vi "Cashew Model.vi"() -> ()   [LabVIEW 2018]
uses:
  <vilib>/express/express arith-compare/Formula/XNode/ExpressFormulaBlockNode.xnode
panel:
  out "Array":dbl[](array[numeric])
  out "Condition Satified?":bool
  out "Waveform Chart":dbl[](graph)
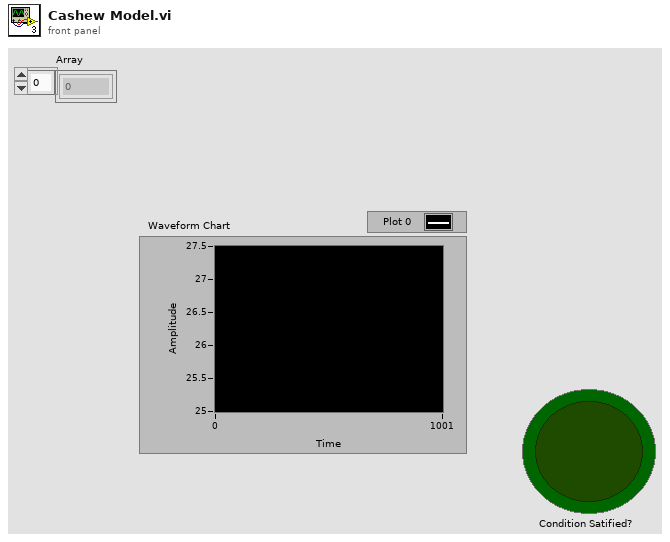
[diagram p1: front panel]
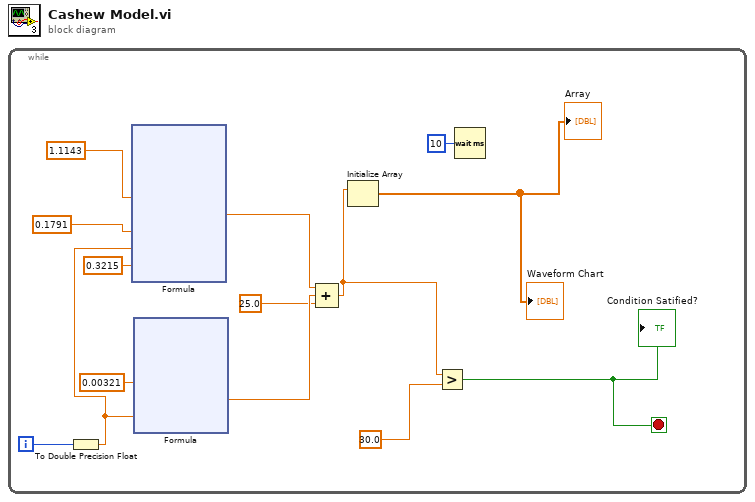
[diagram p0: block diagram]
diagram:
  n1 = while {
    i -> [w14]
    stop <- w4 stop-if-true
    n2 = To Double Precision Float(number=w14) -> (double precision float=w7:dbl)
    n3 = xnode "Formula"("a"=1.1143, "K"=0.1791, "t"=w7, "n"=0.3215) -> ("Result"=w9:dbl)  [unwired: 1 in, 1 out]
    n4 = xnode "Formula"("b"=0.00321, "t"=w7) -> ("Result"=w8:dbl)  [unwired: 1 in, 1 out]
    n5 = Compound Arithmetic op=ADD(w9, w8, 25.0 ("value")) -> (w1:dbl)
    n6 = Initialize Array(w1) -> (→"Waveform Chart" →"Array":dbl[])  [unwired: 1 in]
    n7 = Greater?(x=w1, y=30.0) -> (0:w4:bool)
    "Condition Satified?" <- w4
    n8 = Wait (ms)(milliseconds to wait=u32 10) -> ()  [unwired: 1 out]
  }
